vi "Get Aircraft RC.vi"(8 "Error In":errorcluster, 11 "Aircraft ID":u8) -> (0 "Error Out":errorcluster, 3 "Aircraft RC Data":T1)   [LabVIEW 2014]
uses:
  Controls/Aircraft RC Data.ctl
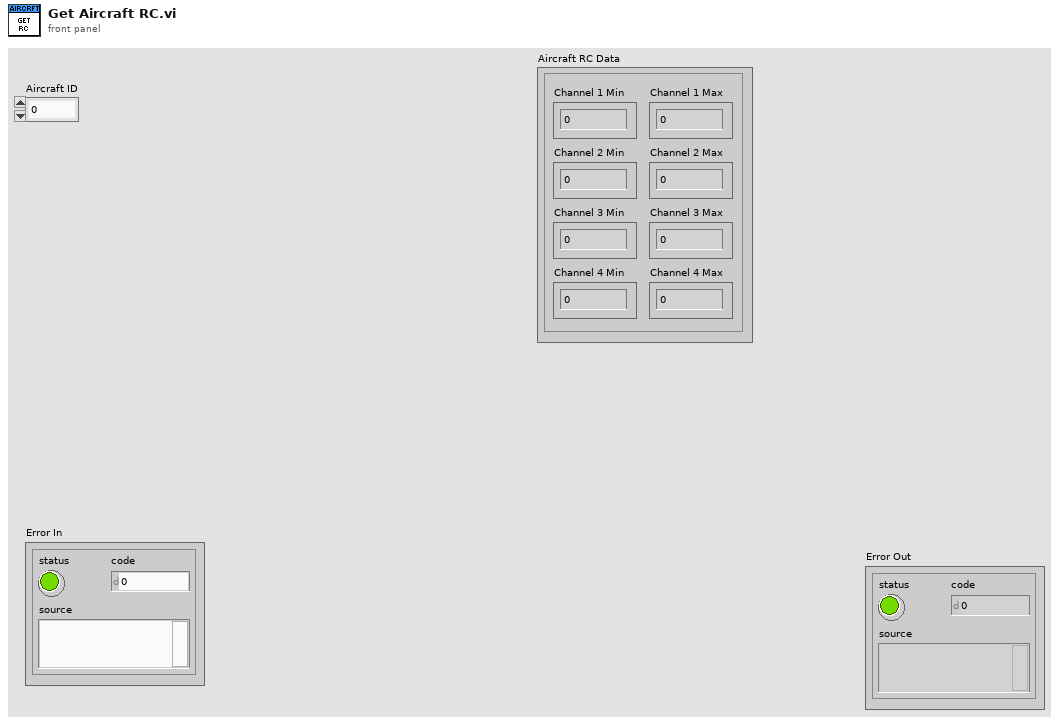
[diagram p1: front panel]
types:
  T1 = typedef "Aircraft RC Data.ctl" = cluster{"Channel 1 Min":i16, "Channel 1 Max":i16, "Channel 2 Min":i16, "Channel 2 Max":i16, "Channel 3 Min":i16, "Channel 3 Max":i16, "Channel 4 Min":i16, "Channel 4 Max":i16}
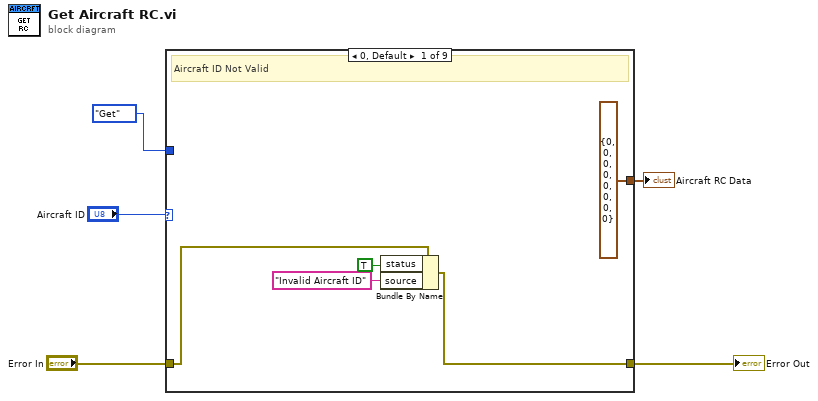
[diagram p0: block diagram]
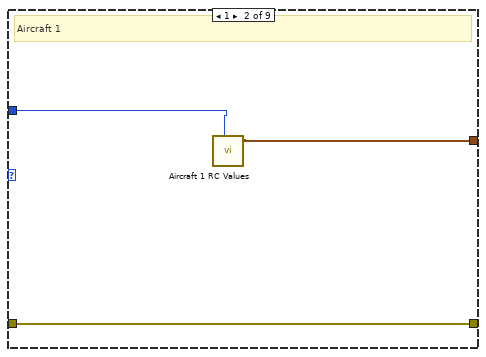
[diagram p2: hidden frame]
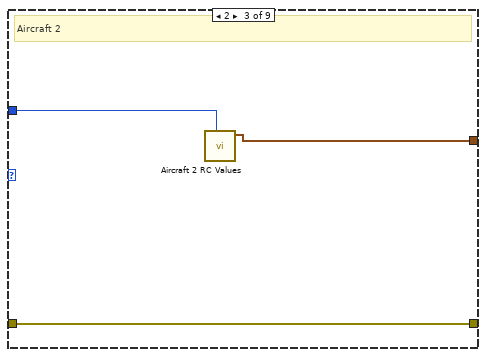
[diagram p3: hidden frame]
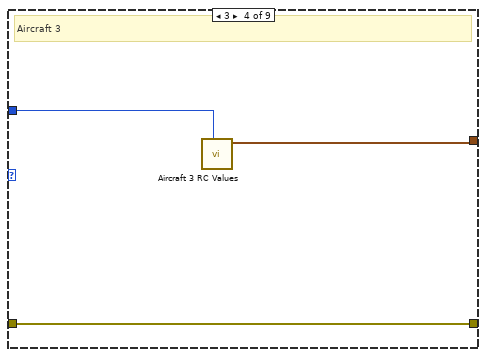
[diagram p4: hidden frame]
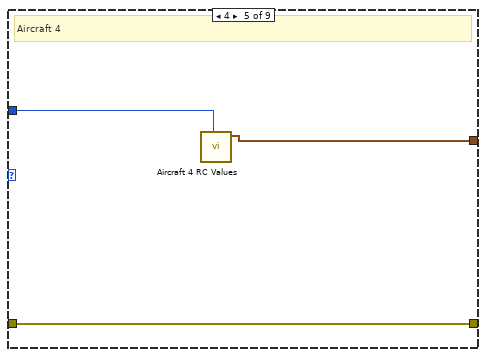
[diagram p5: hidden frame]
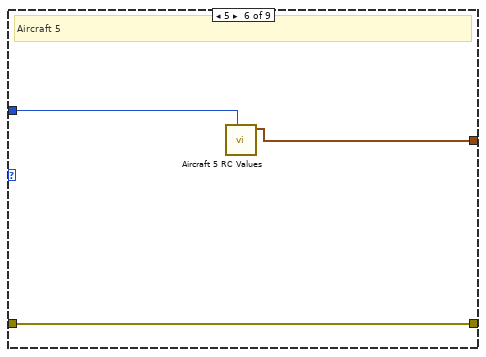
[diagram p6: hidden frame]
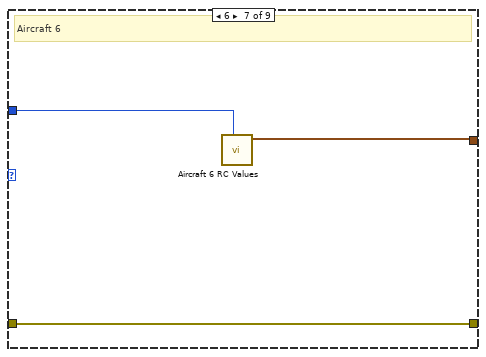
[diagram p7: hidden frame]
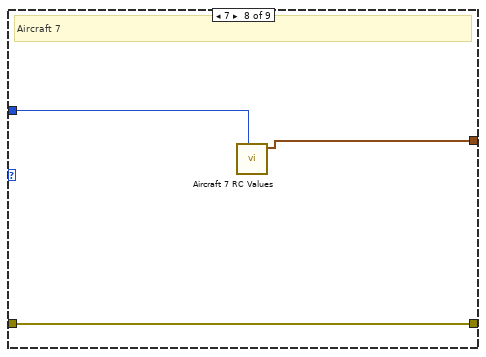
[diagram p8: hidden frame]
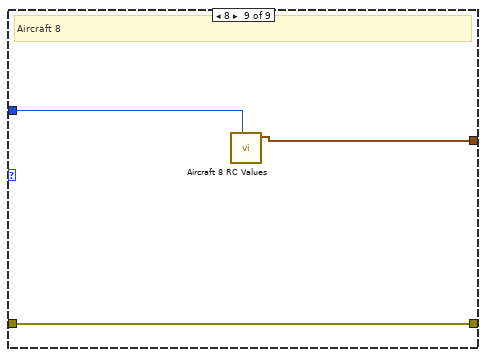
[diagram p9: hidden frame]
diagram:
  n1 = case shown="0, Default" "Aircraft ID" {
    tunnel: [T1 {"Channel 1 Min"=0, "Channel 1 Max"=0, "Channel 2 Min"=0, "Channel 2 Max"=0, "Channel 3 Min"=0, "Channel 3 Max"=0, "Channel 4 Min"=0, "Channel 4 Max"=0} ("Aircraft RC Data 2") w12 w15 w17 w21 w23 w26 w29 w32] -> w1
    tunnel: [w9 w13 w16 w19 w22 w25 w28 w31 w34] -> w4
    tunnel: "Error In" -> [w10 w13 w16 w19 w22 w25 w28 w31 w34]
    tunnel: enum16{"Get", "Set"}."Get" ("Method") -> [_ w11 w14 w18 w20 w24 w27 w30 w33]
    frame 0, Default {
      # "Aircraft ID Not Valid"
      n2 = Bundle By Name(cluster=w10, "status"=TRUE, "source"="Invalid Aircraft ID") -> (w9:errorcluster)
    }
    frame 1 {
      # "Aircraft 1"
      n3 = call "Aircraft 1 RC Values .vi"("Method"=w11) -> ("Aircraft RC Data 2"=w12:T1)  [unwired: 10 in]
    }
    frame 2 {
      # "Aircraft 2"
      n4 = call "Aircraft 2 RC Values .vi"("Method"=w14) -> ("Aircraft RC Data 2"=w15:T1)  [unwired: 10 in]
    }
    frame 3 {
      # "Aircraft 3"
      n5 = call "Aircraft 3 RC Values .vi"("Method"=w18) -> ("Aircraft RC Data 2"=w17:T1)  [unwired: 10 in]
    }
    frame 4 {
      # "Aircraft 4"
      n6 = call "Aircraft 4 RC Values .vi"("Method"=w20) -> ("Aircraft RC Data 2"=w21:T1)  [unwired: 10 in]
    }
    frame 5 {
      # "Aircraft 5"
      n7 = call "Aircraft 5 RC Values .vi"("Method"=w24) -> ("Aircraft RC Data 2"=w23:T1)  [unwired: 10 in]
    }
    frame 6 {
      # "Aircraft 6"
      n8 = call "Aircraft 6 RC Values .vi"("Method"=w27) -> ("Aircraft RC Data 2"=w26:T1)  [unwired: 10 in]
    }
    frame 7 {
      # "Aircraft 7"
      n9 = call "Aircraft 7 RC Values .vi"("Method"=w30) -> ("Aircraft RC Data 2"=w29:T1)  [unwired: 10 in]
    }
    frame 8 {
      # "Aircraft 8"
      n10 = call "Aircraft 8 RC Values .vi"("Method"=w33) -> ("Aircraft RC Data 2"=w32:T1)  [unwired: 10 in]
    }
  }
  "Error Out" <- w4
  "Aircraft RC Data" <- w1
